vi "read_attributes.vi"(8 "error in (no error)":errorcluster caption="entrée d'erreur (pas d'erreur)", 11 "ARDRegression en entrée":refnum<class "ARDRegression.lvclass">) -> (0 "error out":errorcluster caption="sortie d'erreur", 2 "attributes":T1, 3 "ARDRegression en sortie":refnum<class "ARDRegression.lvclass">)   [LabVIEW 2020, in "ARDRegression.lvclass"]
uses:
  ARDRegression.lvclass
  Controls/ardregressor_attributes.ctl
  ARDRegression.lvclass/ARDRegression.ctl
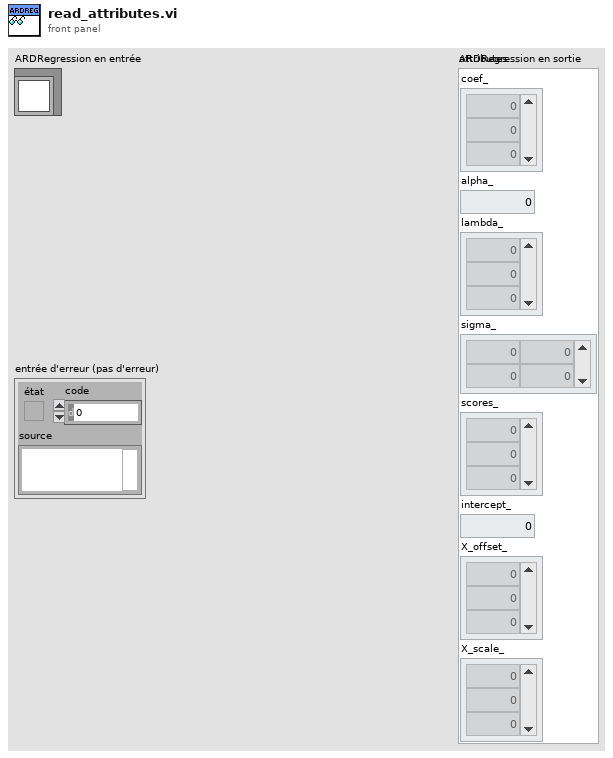
[diagram p1: front panel]
types:
  T1 = typedef "ardregressor_attributes.ctl" = cluster{"coef_":dbl[], "alpha_":dbl, "lambda_":dbl[], "sigma_":dbl[][], "scores_":dbl[], "intercept_":dbl, "X_offset_":dbl[], "X_scale_":dbl[]}
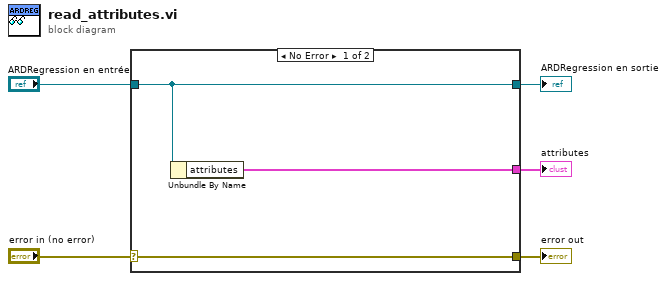
[diagram p0: block diagram]
diagram:
  n1 = case shown="No Error" "error in (no error)" {
    selector: "error in (no error)" -> [w8 w9]
    tunnel: [w8 w9] -> w4
    tunnel: [w7 w10] -> w2
    tunnel: "ARDRegression en entrée" -> [w7 w10]
    tunnel: [w6 _] -> w1
    frame No Error {
      n2 = Unbundle By Name(w7) -> ("attributes"=w6:T1)
    }
    frame Error {
    }
  }
  "error out" <- w4
  "ARDRegression en sortie" <- w2
  "attributes" <- w1
